vi "Parse_Metadata_JSONSTRING.vi"(8 "error in (no error)":errorcluster, 11 "JSON String":string) -> (0 "error out":errorcluster, 1 "Sweep Metadata Cluster":T1 {"Channels: AO"."AO f (Hz)" min=0.001 max=10000.0; "Channels: AO"."AO DC (V)" format="%#_6p"; "Channels: AO"."AO amp (V)" format="%#_6p"}, 2 "parsed info output":T17 {"Sorted scan parameters"."?"."Rate" format="%.2f"; "Sorted scan parameters"."?"."Step" format="%#_6p"; "Sorted scan parameters"."?"."End" format="%#_6p"; "Sorted scan parameters"."?"."Start" format="%#_6p"})   [LabVIEW 2016]
uses:
  levylab_expt_transport/src/SMOs/SweepControl/Typedefs/ScanControl.ctl
  levylab_expt_transport/src/SMOs/SweepControl/Typedefs/Cluster - ScanControl.ctl
  levylab_expt_transport/src/SMOs/SweepControl/Typedefs/Enum - Priority.ctl
  levylab_expt_transport/src/SMOs/SweepControl/Typedefs/Enum - Action.ctl
  levylab_expt_transport/src/SMOs/SweepControl/Typedefs/ScanParamters.ctl
  levylab_expt_transport/src/SMOs/SweepControl/Typedefs/Cluster - ScanParamters.ctl
  levylab_expt_transport/src/subVI/SweepMetadataV2.ctl
  <userlib>/LevyLab/Lockin-Multichannel/Typedefs/AO-cluster.ctl
  <userlib>/LevyLab/Lockin-Multichannel/Typedefs/AO_Amp-array.ctl
  <userlib>/LevyLab/Lockin-Multichannel/Typedefs/AO_DC-array.ctl
  <userlib>/LevyLab/Lockin-Multichannel/Typedefs/AO_f-array.ctl
  <userlib>/LevyLab/Lockin-Multichannel/Typedefs/AO_phi-array.ctl
  <userlib>/LevyLab/Lockin-Multichannel/Typedefs/Function-array.ctl
  <userlib>/LevyLab/Lockin-Multichannel/Typedefs/Function-enum.ctl
  levylab_expt_transport/src/SMOs/SweepControl/Typedefs/PostAction.ctl
  levylab_expt_transport/src/SMOs/SweepControl/Typedefs/Enum - PostAction.ctl
  levylab_expt_transport/src/subVI/SweepMetadata.ctl
  levylab_expt_transport/src/SMOs/SweepControl/SweepControl.lvclass
  <vilib>/addons/_JKI.lib/Serialization/JSON/JKI JSON Serialization.lvlib
panel:
  out "# Of Sweep Pts. Fast to Slow":i16[](array[numeric])
  out "Sorted scan parameters":cluster{T15}[](array[cluster])=[{[{"DAQ Channel"=2, "Label"="\nscaledVsg1=", "Start"=0.14, "End"=-0.060000000000000005, "Step"=-0.060000000000000005, "Rate"=0.0, "VISA resource name"="", "wait (ms)"=10000}]}, {[{"DAQ Channel"=2, "Label"="\nscaledVsg1=", "Start"=0.14, "End"=-0.060000000000000005, "Step"=-0.060000000000000005, "Rate"=0.0, "VISA resource name"="", "wait (ms)"=10000}]}, {[{"DAQ Channel"=2, "Label"="\nscaledVsg1=", "Start"=0.14, "End"=-0.060000000000000005, "Step"=-0.060000000000000005, "Rate"=0.0, "VISA resource name"="", "wait (ms)"=10000}, {"DAQ Channel"=3, "Label"="\nscaledVsg1=", "Start"=0.14, "End"=-0.060000000000000005, "Step"=-0.060000000000000005, "Rate"=0.0, "VISA resource name"="", "wait (ms)"=10000}]}] {"?"."Rate" format="%.2f"; "?"."Step" format="%#_6p"; "?"."End" format="%#_6p"; "?"."Start" format="%#_6p"}
  out "Sorted scan control":cluster{T11}[](array[cluster])=[{[{"Priority"=enum."Priority 0", "Scan name"=enum."DSA_Vsg2"}]}, {[{"Priority"=enum."Priority 1", "Scan name"=enum."DSA_Vamp"}]}, {[{"Priority"=enum."Priority 2", "Scan name"=enum."DSA_Vsg1"}, {"Priority"=enum."Priority 2", "Scan name"=enum."DSA_Vsg3"}]}]
  # "1st = # of lowest number priority = highest priority"
  # "0"
  # "1"
  # "2"
  # "3"
  # "4"
  # "5"
  # "6"
  # "7"
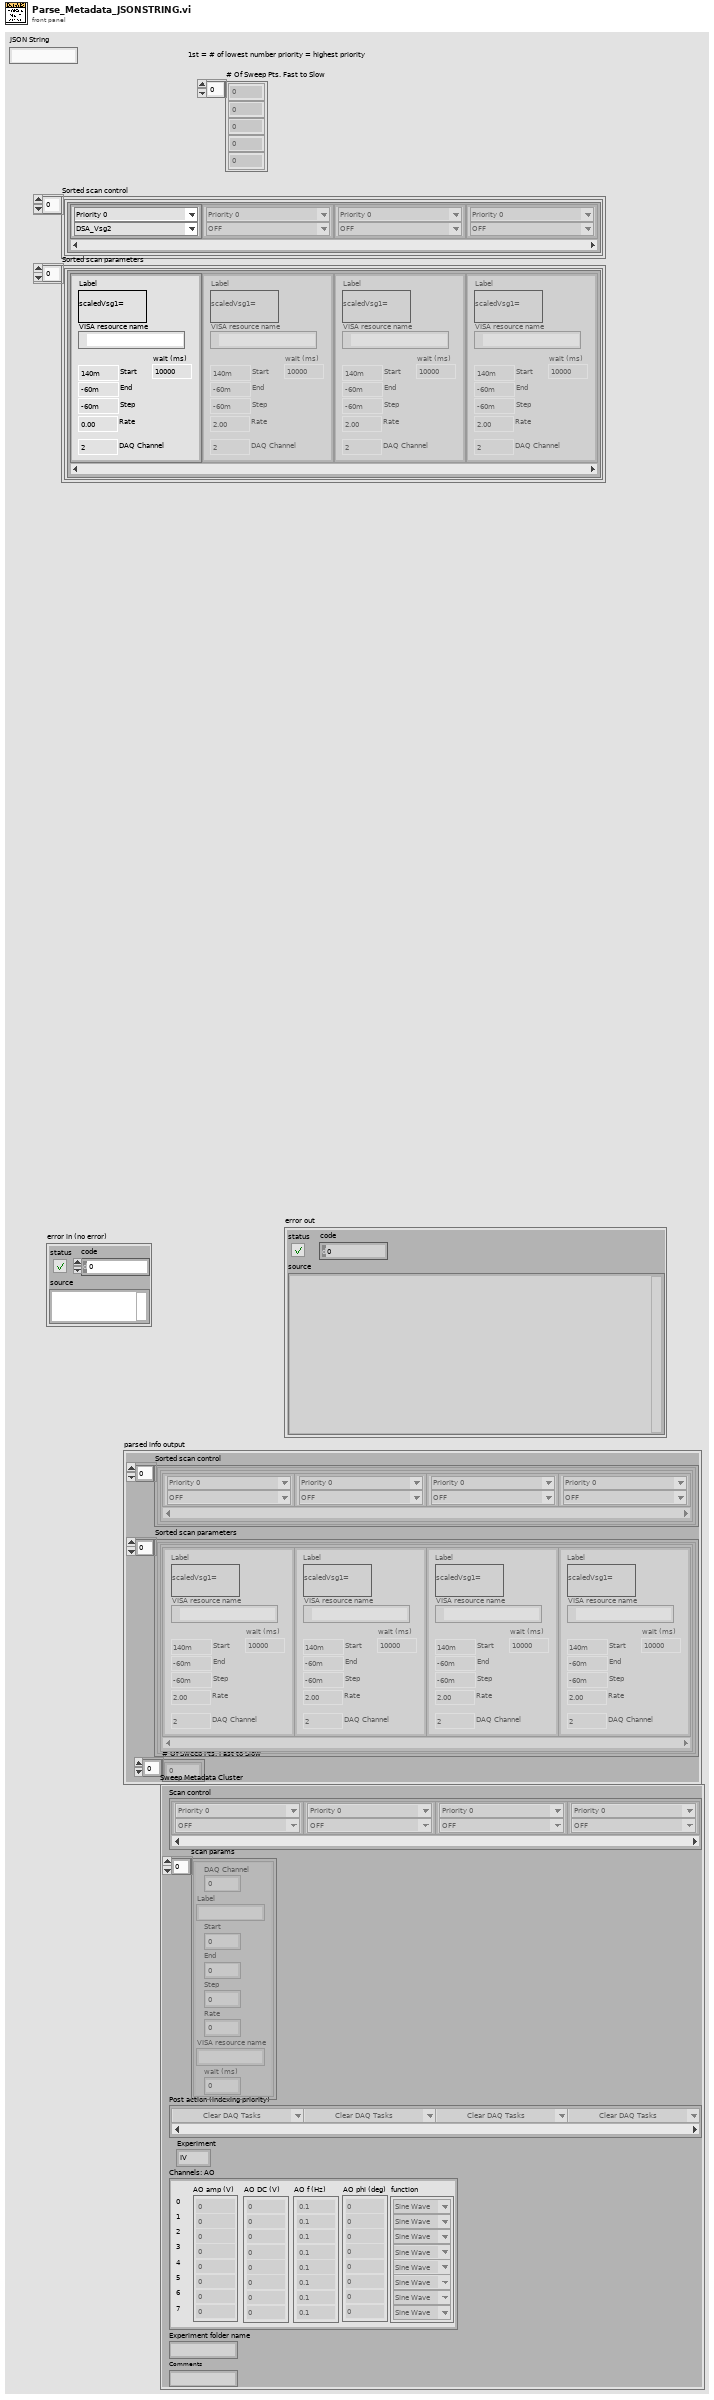
[diagram p1: front panel]
types:
  T1 = typedef "SweepMetadataV2.ctl" = cluster{"Experiment":enum16{"IV", "lockin_time", "Lockin_Vsg"}, "Experiment folder name":string, "Comments":string, "Channels: AO":T2, "Post action (indexing priority)":T9, "Scan control":T11, "scan params":cluster{"DAQ Channel":i32, "Label":string, "Start":dbl, "End":dbl, "Step":dbl, "Rate":dbl, "VISA resource name":string, "wait (ms)":u32}[]}
  T2 = typedef "AO-cluster.ctl" = cluster{"AO amp (V)":T3, "AO DC (V)":T4, "AO f (Hz)":T5, "AO phi (deg)":T6, "function":T7}
  T3 = typedef "AO_Amp-array.ctl" = dbl[]
  T4 = typedef "AO_DC-array.ctl" = dbl[]
  T5 = typedef "AO_f-array.ctl" = dbl[]
  T6 = typedef "AO_phi-array.ctl" = dbl[]
  T7 = typedef "Function-array.ctl" = T8[]
  T8 = typedef "Function-enum.ctl" = enum16{"Sine Wave", "Triangle Wave", "Square Wave", "Sawtooth Wave"}
  T9 = typedef "SweepControl.lvclass/PostAction.ctl" = T10[]
  T10 = typedef "SweepControl.lvclass/Enum - PostAction.ctl" = enum16{"Clear DAQ Tasks", "Check Temperature", "Wait", "Do Nothing"}
  T11 = typedef "SweepControl.lvclass/ScanControl.ctl" = T12[]
  T12 = typedef "SweepControl.lvclass/Cluster - ScanControl.ctl" = cluster{"Priority":T13, "Scan name":T14}
  T13 = typedef "SweepControl.lvclass/Enum - Priority.ctl" = enum16{"Priority 0", "Priority 1", "Priority 2", "Priority 3", "Priority 4", "Priority 5"}
  T14 = typedef "SweepControl.lvclass/Enum - Action.ctl" = enum16{"OFF", "DSA_Vamp", "DSA_freq", "DSA_Vsg1", "DSA_Vsg2", "DSA_Vsg3", "DAQ_Vbg", "B_Field", "Humidity", "Temp", "MW_freq1", "MW_freq2", "MW_amplitude1", "MW_amplitude2"}
  T15 = typedef "SweepControl.lvclass/ScanParamters.ctl" = T16[]
  T16 = typedef "SweepControl.lvclass/Cluster - ScanParamters.ctl" = cluster{"DAQ Channel":i32, "Label":string, "Start":dbl, "End":dbl, "Step":dbl, "Rate":dbl, "VISA resource name":refnum<visa-resource-name>, "wait (ms)":u32}
  T17 = cluster{"Sorted scan control":cluster{T11}[], "Sorted scan parameters":cluster{T15}[], "# Of Sweep Pts. Fast to Slow":i16[]}
  T18 = typedef "SweepMetadata.ctl" = cluster{"Scan control":T11, "Scan Parameters":cluster{"DAQ Channel":i32, "Label":string, "Start":dbl, "End":dbl, "Step":dbl, "Rate":dbl, "VISA resource name":string, "wait (ms)":u32}[], "Post action (indexing priority)":T9, "Experiment":enum16{"IV", "lockin_time", "Lockin_Vsg"}, "Channels: AO":T2, "Experiment folder name":string, "Comments":string}
  T19 = cluster{"Experiment":enum16{"IV", "lockin_time", "Lockin_Vsg"}, "Experiment folder name":string, "Comments":string, "Channels: AO":T2, "Post action (indexing priority)":T9, "Scan control":T11, "scan params":cluster{"DAQ Channel":i32, "Label":string, "Start":dbl, "End":dbl, "Step":dbl, "Rate":dbl, "wait (ms)":u32, "visa resource name":string}[]}
  T20 = cluster{"Sorted scan control":cluster{T11}[], "Sorted scan parameters":cluster{T15}[], i16[]}
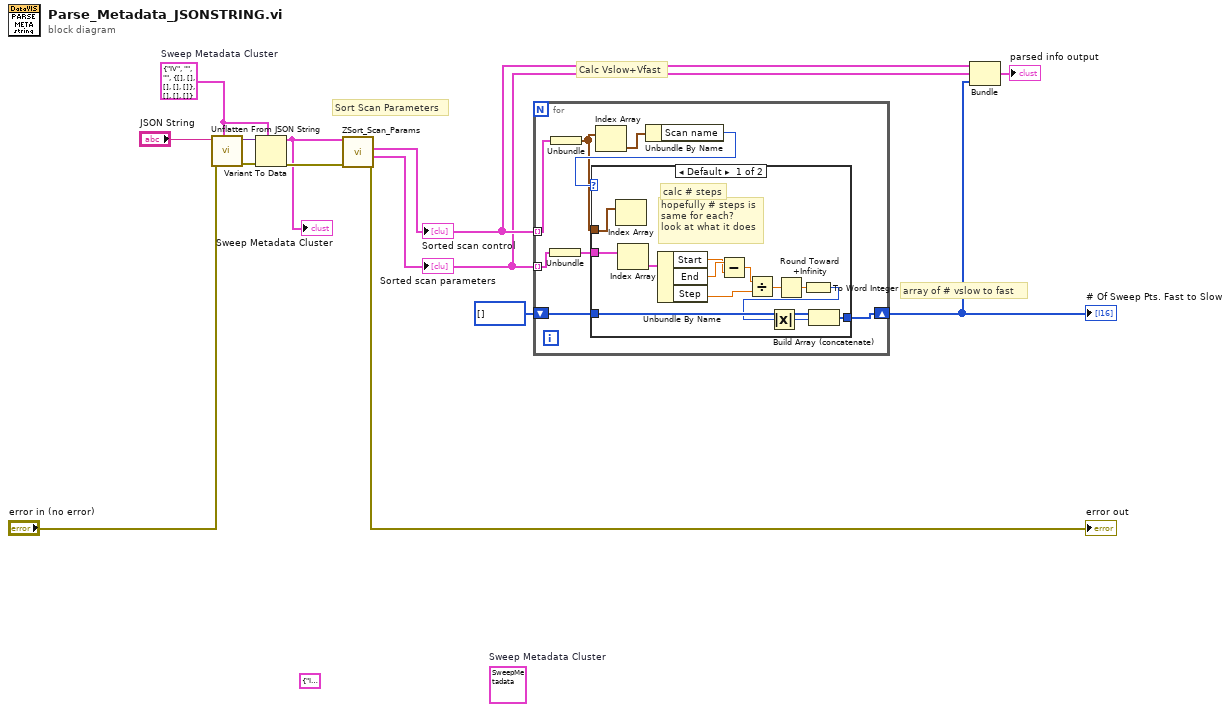
[diagram p0: block diagram]
diagram:
  w5 = T1 {"Experiment"=enum."IV", "Experiment folder name"="", "Comments"="", "Channels: AO"={"AO amp (V)"=[], "AO DC (V)"=[], "AO f (Hz)"=[], "AO phi (deg)"=[], "function"=[]}, "Post action (indexing priority)"=[], "Scan control"=[], "scan params"=[]}  # Sweep Metadata Cluster
  (unwired) T18 {"Scan control"=[], "Scan Parameters"=[], "Post action (indexing priority)"=[], "Experiment"=enum."IV", "Channels: AO"={"AO amp (V)"=[], "AO DC (V)"=[], "AO f (Hz)"=[], "AO phi (deg)"=[], "function"=[]}, "Experiment folder name"="", "Comments"=""}  # Sweep Metadata Cluster
  (unwired) T19 {"Experiment"=enum."IV", "Experiment folder name"="", "Comments"="", "Channels: AO"={"AO amp (V)"=[], "AO DC (V)"=[], "AO f (Hz)"=[], "AO phi (deg)"=[], "function"=[]}, "Post action (indexing priority)"=[], "Scan control"=[], "scan params"=[]} ("output cluster 2")
  # "array of # vslow to fast"
  # "Calc Vslow+Vfast"
  # "Sort Scan Parameters"
  n1 = call <vilib>:"Unflatten From JSON String.vi"("Type and Defaults"=w5, "error in (no error)"="error in (no error)", "JSON String"="JSON String") -> ("error out"=w12:errorcluster, "Variant"=w13:variant)  [unwired: 7 in]
  n2 = Variant To Data(error in=w12, type=w5, Variant=w13) -> (data=w4:T1, error out=w11:errorcluster)
  "Sweep Metadata Cluster" <- w4
  n3 = call "ZSort_Scan_Params.vi"("error in (no error)"=w11, "Sweep Metadata Cluster"=w4) -> ("error out"=→"error out":errorcluster, "Sorted scan parameters"=w8:cluster{T15}[], "Sorted scan control"=w9:cluster{T11}[])  [unwired: 7 in]
  "Sorted scan control" <- w9
  "Sorted scan parameters" <- w8
  n4 = for {
    tunnel: w9 -> [w21] mode=indexing
    tunnel: w8 -> [w17] mode=indexing
    shift-right: [w14] -> w7
    shift-left: i16[] [] -> [w15]
    n5 = Unbundle(w17) -> (w16:T15)
    n6 = Unbundle(w21) -> (w18:T11)
    n7 = Index Array(array=w18) -> (element=w20:T12)  [unwired: 1 in]
    n8 = Unbundle By Name(w20) -> ("Scan name"=w19:T14)
    n9 = case shown="Default" w19 {
      tunnel: w18 -> [w34 _]
      tunnel: w16 -> [w33 _]
      tunnel: w15 -> [w27 w35]
      tunnel: [w26 w35] -> w14
      frame Default {
        # "hopefully # steps is\nsame for each?\nlook at what it does"
        # "calc # steps"
        n10 = Index Array(array=w34) -> ()  [unwired: 1 in, 1 out]
        n11 = Index Array(array=w33) -> (element=w32:T16)  [unwired: 1 in]
        n12 = Unbundle By Name(w32) -> ("Start"=w30:dbl, "End"=w31:dbl, "Step"=w28:dbl)
        n13 = Subtract(x=w31, y=w30) -> (x-y=w29:dbl)
        n14 = Divide(x=w29, y=w28) -> (x/y=w25:dbl)
        n15 = Round Toward +Infinity(x=w25) -> (ceil(x): smallest int >= x=w24:dbl)
        n16 = To Word Integer(number=w24) -> (16bit integer=w23:i16)
        n17 = Absolute Value(x=w23) -> (abs(x)=w22:i16)
        n18 = Build Array (concatenate)(w27, w22) -> (w26:i16[])
      }
      frame "OFF" {
        # "Ignore this one"
      }
    }
  }
  "# Of Sweep Pts. Fast to Slow" <- w7
  n19 = Bundle("Sorted scan control"=w9, "Sorted scan parameters"=w8, w7) -> (→"parsed info output":T20)  [unwired: 1 in]
